vi "断电保存全局.vi"() -> ()   [LabVIEW 2016]
panel:
  in  "拆分间隔(默认100)":i32=100
  in  "url":string="127.0.0.1:1000"
  in  "equipmentCode":string="AH CODCR"
  in  "time":string="2021-05-08 14:02:02"
  in  "data path":path=path "C:/Users/TinkPad/Desktop/光谱数据"
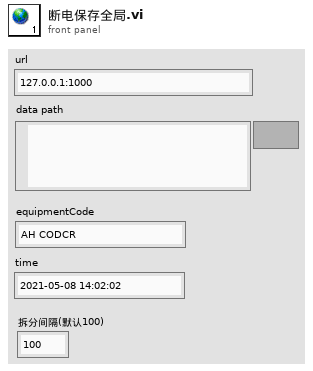
[diagram p1: front panel]
diagram:
